vi "Message Popup.vi"(8 "error in":errorcluster, 10 "Message":string) -> (0 "error out":errorcluster, 2 "Cancel Button out":bool, 3 "OK Button out":bool)   [LabVIEW 2022 SP3]
panel:
  in  "Cancel Button":bool
  in  "OK Button":bool
  out "Display":string
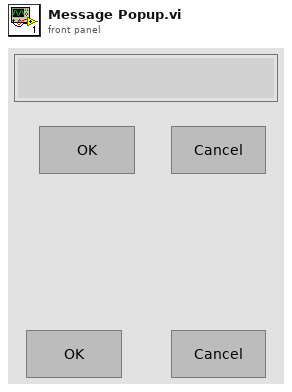
[diagram p1: front panel]
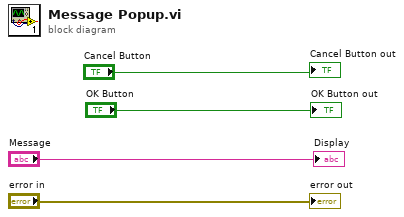
[diagram p0: block diagram]
diagram:
  "Display" <- "Message"
  "error out" <- "error in"
  "Cancel Button out" <- "Cancel Button"
  "OK Button out" <- "OK Button"
